vi "SetExplicitMessage_lowlevel.vi"(6 "value":u8[](array[numeric]), 7 "Class":i32, 8 "error in (no error)":errorcluster, 9 "Attribute":i32, 10 "assembly instance ID":u32, 11 ".NET Refnum in":refnum<k24>) -> (0 "error out":errorcluster, 1 "SetAttributeSingle":u8[](array[numeric]), 2 "Numeric":i32, 3 ".NET Refnum out":refnum<k24>)   [LabVIEW 2022 SP3, in "Motor Controller.lvclass"]
uses:
  Motor Controller.lvclass
  C:/projects/Digilens_IPLC2/Classes/Motor Controller/EEIP.dll
  EEIP.dll
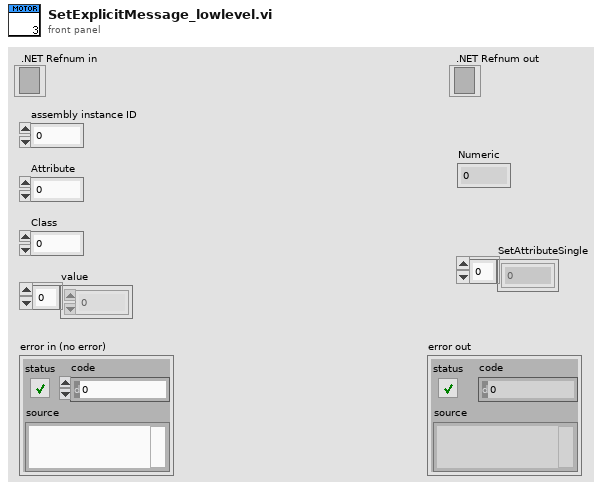
[diagram p1: front panel]
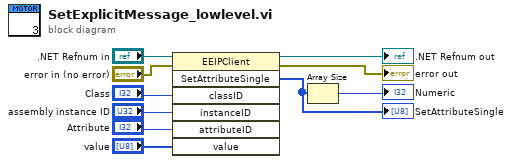
[diagram p0: block diagram]
diagram:
  n1 = invoke class="EEIPClient" method="SetAttributeSingle"(reference=".NET Refnum in", error in="error in (no error)", "classID"="Class", "instanceID"="assembly instance ID", "attributeID"="Attribute", "value"="value") -> (reference out=→".NET Refnum out":refnum<k24>, error out=→"error out":errorcluster, "SetAttributeSingle"=w5:u8[])  [unwired: 1 in, 4 out]
  "SetAttributeSingle" <- w5
  n2 = Array Size(array=w5) -> (size(s)=→"Numeric":i32)
